vi "CRYGraph Property Window Picture.vi"(8 "Tab Name":string, 9 "Graph VI Ref":refnum<vi>) -> ()   [LabVIEW 2013]
uses:
  Control/CRYPicture Property.ctl
panel:
  in  "Picture Property":T1
  in  "OK":bool
  in  "Picture Tab":enum32{"Title", "Picture"}(tab)
  in  "Title Name":string caption="标题名字"
  in  "Show vertical scroll bar":bool caption="显示垂直滚动条"
  in  "Show horizontal scroll bar":bool caption="显示水平滚动条"
  in  "Browse":bool
  in  "Image Path":string caption="图片路径"
  in  "Resize Picture to Window":bool
  in  "Resize Window to Picture":bool
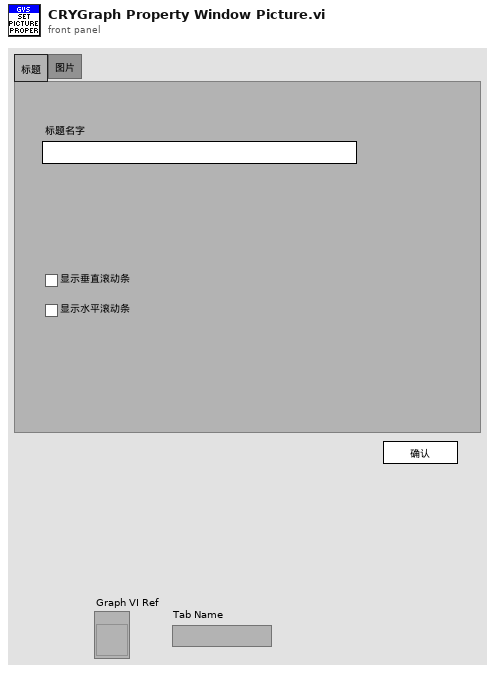
[diagram p1: front panel]
types:
  T1 = typedef "CRYPicture Property.ctl" = cluster{"Image Path":string, "Show vertical scroll bar":bool, "Show horizontal scroll bar":bool}
  T2 = enum16{"Left Button", "Center Button", "Right Button", "Window Close"}
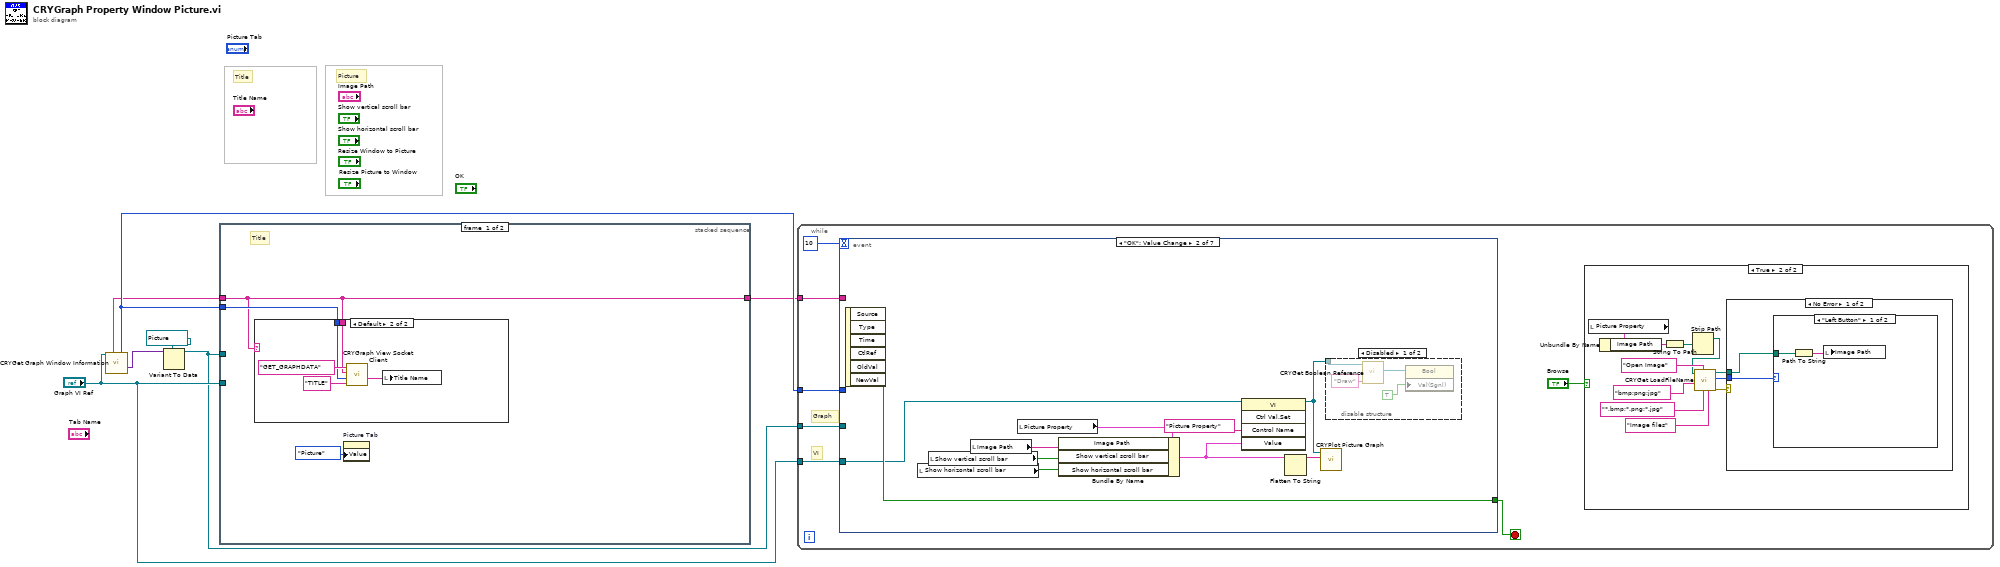
[diagram p0: block diagram]
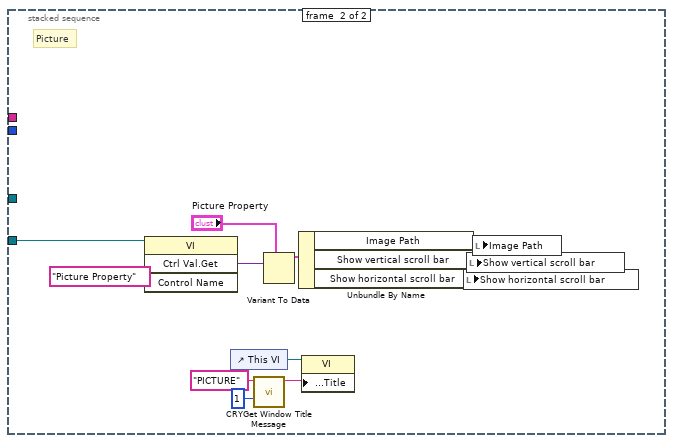
[diagram p3: hidden frame]
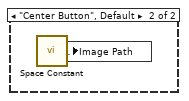
[diagram p5: hidden frame]
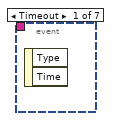
[diagram p7: hidden frame]
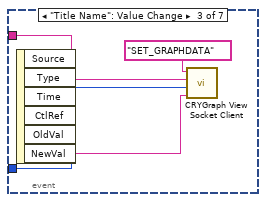
[diagram p9: hidden frame]
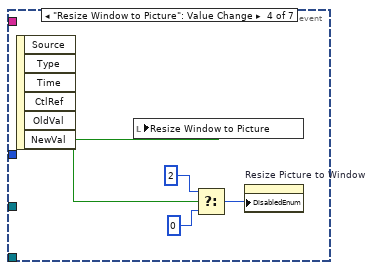
[diagram p10: hidden frame]
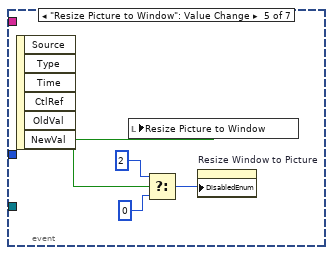
[diagram p11: hidden frame]
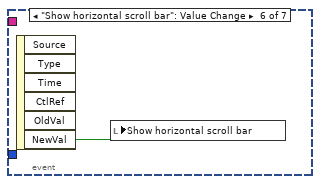
[diagram p12: hidden frame]
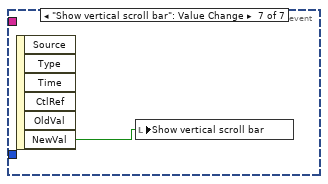
[diagram p13: hidden frame]
diagram:
  # "Title"
  # "Picture"
  n1 = call "CRYGet Graph Window Information.vi"("pGraph VI In"="Graph VI Ref") -> ("Queue Name Out"=w5:string, "Graph Number Out"=w6:i32, "Graph Control Ref Out"=w1:variant)  [unwired: 2 in, 10 out]
  n2 = Variant To Data(type=refnum<vi> refnum ("XY Graph"), Variant=w1) -> (data=w3:refnum<vi>)  [unwired: 1 in, 1 out]
  n3 = stacked-sequence {
    tunnel: "Graph VI Ref" -> [_ w27]
    tunnel: w6 -> [w10 _]
    tunnel: w5 -> [w9 _]
    tunnel: [w9 _] -> w4
    tunnel: w3 -> [_ _]
    frame #0 {
      # "Title"
      n4 = case shown="Default" w9 {
        tunnel: w10 -> [_ w13]
        tunnel: w9 -> [_ w12]
        frame "test DataView" {
        }
        frame Default {
          n5 = call "CRYGraph View Socket Client.vi"("sOption"="TITLE", "nData"=w13, "sData"=w12, "sAction"="GET_GRAPHDATA") -> ("sData Out"=w11:string)  [unwired: 4 in, 3 out]
          n6 = local write "Title Name"(w11) -> ()
        }
      }
      n7 = property on="Picture Tab" class="TabCtl (strict)"("Value"=enum32{"Title", "Picture"}."Picture" ("Tab Control")) -> ()  [unwired: 2 in, 2 out]
    }
    frame #1 {
      # "Picture"
      n8 = invoke class="VI" method="Ctrl Val.Get"(reference=w27, "Control Name"="Picture Property") -> ("Get Control Value Variant"=w25:variant)  [unwired: 2 in, 3 out]
      n9 = control-ref of="This VI"() -> (w16:refnum<vi>)
      n10 = call "CRYGet Window Title Message.vi"("No"=1 ("Error No"), "Kind"="PICTURE") -> ("Multibyte String"=w17:string)  [unwired: 4 in, 5 out]
      n11 = Variant To Data(type="Picture Property", Variant=w25) -> (data=w23:T1)  [unwired: 1 in, 1 out]
      n12 = Unbundle By Name(w23) -> ("Image Path"=w22:string, "Show vertical scroll bar"=w21:bool, "Show horizontal scroll bar"=w20:bool)
      n13 = property class="VI"(reference=w16, "Front Panel.Title"=w17) -> ()  [unwired: 1 in, 2 out]
      n14 = local write "Show horizontal scroll bar"(w20) -> ()
      n15 = local write "Show vertical scroll bar"(w21) -> ()
      n16 = local write "Image Path"(w22) -> ()
    }
  }
  n17 = while {
    tunnel: w6 -> [w33]
    tunnel: "Graph VI Ref" -> [w32]
    tunnel: w4 -> [w29]
    tunnel: w3 -> [w28]
    stop <- w31 stop-if-true
    # "Graph"
    # "VI"
    n18 = event shown="[1] \"OK\": Value Change" {
      selector: _ -> [_ _ _ _ _ _ _]
      dyn-events: _ -> [_ _ _ _ _ _ _]
      timeout: 10 -> [_ _ _ _ _ _ _]
      tunnel: [_ w60 _ _ _ _ _] -> w31
      tunnel: w33 -> [_ _ w65 _ _ _ _]
      tunnel: w32 -> [_ w59 _ _ _ _ _]
      tunnel: w29 -> [_ _ w67 _ _ _ _]
      tunnel: w28 -> [_ _ _ _ _ _ _]
      event Timeout {
        n19 = event-data() -> ()  [unwired: 3 out]
      }
      event "OK": Value Change {
        n20 = event-data() -> ("NewVal"=w60:bool)  [unwired: 6 out]
        n21 = local read "Show horizontal scroll bar"() -> (w52:bool)
        n22 = local read "Show vertical scroll bar"() -> (w53:bool)
        n23 = local read "Image Path"() -> (w54:string)
        n24 = local read "Picture Property"() -> (w56:T1)
        n25 = Bundle By Name(cluster=w56, "Image Path"=w54, "Show vertical scroll bar"=w53, "Show horizontal scroll bar"=w52) -> (w57:T1)
        n26 = invoke class="VI" method="Ctrl Val.Set"(reference=w59, "Control Name"="Picture Property", "Value"=w57) -> (reference out=w58:refnum<vi>)  [unwired: 2 in, 4 out]
        n27 = Flatten To String(anything=w57) -> (data string=w51:string)  [unwired: 3 in, 2 out]
        n28 = call "CRYPlot Picture Graph.vi"("Flattened Property"=w51, "pGraph VI In"=w58) -> ()  [unwired: 10 in]
        n29 = disable-structure shown="Disabled" {
          disable-tunnel: w58 -> [w64 _]
          frame Disabled {
            n30 = call "CRYGet Boolean Reference.vi"("Label Name"="Draw", "VI Refnum"=w64) -> ("Boolean Ref"=w62:refnum<vi>)  [unwired: 7 in, 2 out]
            n31 = property class="Bool"(reference=w62, "Val(Sgnl)"=TRUE) -> ()  [unwired: 1 in, 2 out]
          }
          frame Enabled {
          }
        }
      }
      event "Title Name": Value Change {
        n32 = event-data() -> ("NewVal"=w66:string)  [unwired: 6 out]
        n33 = call "CRYGraph View Socket Client.vi"("sOption"=w66, "nData"=w65, "sData"=w67, "sAction"="SET_GRAPHDATA") -> ()  [unwired: 4 in, 4 out]
      }
      event "Resize Window to Picture": Value Change {
        n34 = event-data() -> ("NewVal"=w70:bool)  [unwired: 6 out]
        n35 = local write "Resize Window to Picture"(w70) -> ()
        n36 = Select(t=2, s=w70, f=0) -> (s? t:f=w69:i32)
        n37 = property on="Resize Picture to Window" class="Bool (strict)"("DisabledEnum"=w69) -> ()  [unwired: 2 in, 2 out]
      }
      event "Resize Picture to Window": Value Change {
        n38 = event-data() -> ("NewVal"=w74:bool)  [unwired: 6 out]
        n39 = local write "Resize Picture to Window"(w74) -> ()
        n40 = Select(t=2, s=w74, f=0) -> (s? t:f=w73:i32)
        n41 = property on="Resize Window to Picture" class="Bool (strict)"("DisabledEnum"=w73) -> ()  [unwired: 2 in, 2 out]
      }
      event "Show horizontal scroll bar": Value Change {
        n42 = event-data() -> ("NewVal"=w77:bool)  [unwired: 6 out]
        n43 = local write "Show horizontal scroll bar"(w77) -> ()
      }
      event "Show vertical scroll bar": Value Change {
        n44 = event-data() -> ("NewVal"=w78:bool)  [unwired: 6 out]
        n45 = local write "Show vertical scroll bar"(w78) -> ()
      }
    }
    n46 = case shown="True" "Browse" {
      frame False {
      }
      frame True {
        n47 = local read "Picture Property"() -> (w36:T1)
        n48 = Unbundle By Name(w36) -> ("Image Path"=w38:string)
        n49 = String To Path(string=w38) -> (path=w37:path)
        n50 = Strip Path(path=w37) -> (stripped path=w35:path)  [unwired: 1 out]
        n51 = call "CRYGet LoadFileName.vi"("pattern label"="Image files", "pattern (all files)"="*.bmp;*.png;*.jpg", "TitleName"="Open Image" ("Prompt"), "Category Name"="bmp;png;jpg" ("pattern (all files)"), "Start path"=w35) -> ("error out"=w41:errorcluster, "Which Button?"=w45:T2, "Path"=w42:path)  [unwired: 3 in, 1 out]
        n52 = case shown="No Error" w41 {
          tunnel: w45 -> [w47 _]
          tunnel: w42 -> [w46 _]
          frame No Error {
            n53 = case shown="\"Left Button\"" w47 {
              tunnel: w46 -> [w49 _]
              frame "Left Button" {
                n54 = Path To String(path=w49) -> (string=w48:string)
                n55 = local write "Image Path"(w48) -> ()
              }
              frame "Center Button", Default {
                n56 = call <vilib>:"Space Constant.vi"() -> ("String"=w50:string)
                n57 = local write "Image Path"(w50) -> ()
              }
            }
          }
          frame Error {
          }
        }
      }
    }
  }
